vi "GUI_Single Button Pump.vi"() -> ()   [LabVIEW 2011] (continued)
      tunnel: [w32 w122 w128 w148 w153 w159 w162 T20 {"Isolate HPBD"=FALSE, "Core"={"Current VI Reference"=refnum, "Close Panel on Exit?"=FALSE}, "Status Display Array"=[], "Connection URLs"={"Source_URL EC"="", "Target_URL EC"="", "Source_URL LB"="", "Target_URL LB"=""}, "EC Status"={"bits 2"=[], "bits 2"=[], "bits 2"=[], [], "FLOAT NUMBERS 2"=[]}, "EC Status Named"={"EC statusboolarray2"={"Spare 1"=FALSE, "Spare 2"=FALSE, "Spare 3"=FALSE, "Spare 4"=FALSE, "ROUGHING PUMP run opened"=FALSE, "ROUGHING PUMP no fault closed"=FALSE, "BACKING PUMP run opened"=FALSE, "BACKING PUMP no fault closed"=FALSE, "BTL TURBO turbo fault feedback"=FALSE, "BTL TURBO turbo normal feedback"=FALSE, "TARGET 1 TURBO turbo fault feedback"=FALSE, "TARGET 1 TURBO turbo normal feedback"=FALSE, "TARGET 2 TURBO turbo fault feedback"=FALSE, "TARGET 2 TURBO turbo normal feedback"=FALSE, "BTL2 TURBO turbo fault feedback"=FALSE, "BTL2 TURBO turbo normal feedback"=FALSE, "HPD TURBO turbo fault feedback"=FALSE, "HPD TURBO turbo normal feedback"=FALSE, "Spare 5"=FALSE, "Spare 6"=FALSE, "ROUGHING PUMP FLOW SWITCH"=FALSE, "BACKING PUMP FLOW SWITCH"=FALSE, "BTL TURBO FLOW SWITCH"=FALSE, "TARGET 1 TURBO FLOW SWITCH"=FALSE, "TARGET 2 TURBO FLOW SWITCH"=FALSE, "BTL2 TURBO FLOW SWITCH"=FALSE, "HPD TURBO FLOW SWITCH"=FALSE, "Spare 7"=FALSE, "BTL ion gauge on signal"=FALSE, "BTL ion gauge degas signal"=FALSE, "TARGET ion gauge on signal"=FALSE, "TARGET ion gauge degas signal"=FALSE, "BTL2 ion gauge on signal"=FALSE, "BTL2 ion gauge degas signal"=FALSE, "HPD ion gauge on signal"=FALSE, "HPD ion gauge degas signal"=FALSE, "Spare 8"=FALSE, "Spare 9"=FALSE, "Spare 10"=FALSE, "Spare 11"=FALSE, "ROUGHING MANIFOLD VALVE"=FALSE, "BACKING MANIFOLD VALVE"=FALSE, "ROUGHING BACKING CONNECT VALVE"=FALSE, "BTL ROUGHING VALVE"=FALSE, "BTL VENT VALVE"=FALSE, "BTL Turbo Gate Valve"=FALSE, "BTL Turbo Backing Valve"=FALSE, "Roughing Manifold VV"=FALSE, "Backing Manifold VV"=FALSE, "TARGET ROUGHING VALVE"=FALSE, "BTL2 ROUGHING VALVE"=FALSE, "HPD ROUGHING VALVE"=FALSE, "GV BTL-TARGET"=FALSE, "GV TARGET-BTL2"=FALSE, "GV BTL2-HPD"=FALSE, "TARGET VENT VALVE"=FALSE, "BTL2 VENT VALVE"=FALSE, "HPD VENT VALVE"=FALSE, "TARGET  Turbo Gate Valve 1"=FALSE, "TARGET  Turbo Gate Valve 2"=FALSE, "BTL2 Turbo Gate Valve"=FALSE, "HPD  Turbo Gate Valve"=FALSE, "TARGET Turbo Backing Valve 1"=FALSE, "TARGET Turbo Backing Valve 2"=FALSE}, "EC statusboolarray3"={"BTL2 Turbo Backing Valve"=FALSE, "HPD Turbo Backing Valve"=FALSE, "Spare 1"=FALSE, "Spare 2"=FALSE, "Spare 3"=FALSE, "Spare 4"=FALSE, "Spare 5"=FALSE, "Spare 6"=FALSE, "Spare 7"=FALSE, "Spare 8"=FALSE, "Spare 9"=FALSE, "BTL Turbo Vent Valve"=FALSE, "TARGET1 Turbo Vent Valve"=FALSE, "TARGET2 Turbo Vent Valve"=FALSE, "BTL2 Turbo Vent Valve"=FALSE, "HPD Turbo Vent Valve"=FALSE, "Spare 10"=FALSE, "Spare 11"=FALSE, "BTL turbo pump run signal"=FALSE, "TARGET1 turbo pump run signal"=FALSE, "TARGET2 turbo pump run signal"=FALSE, "BTL2 turbo pump run signal"=FALSE, "HPD turbo pump run signal"=FALSE, "Spare 12"=FALSE, "watch dog timer - out"=FALSE, "BTL vented – out"=FALSE, "BTL medvac – out"=FALSE, "BTL hivac – out"=FALSE, "GPM EC - out"=FALSE, "GVM EC - out"=FALSE, "RP EC status - out"=FALSE, "RP LB toggle - out"=FALSE, "GATE ALL - closed out"=FALSE, "Spare 13"=FALSE, "Spare 14"=FALSE, "Spare 15"=FALSE, "Spare 16"=FALSE, "Spare 17"=FALSE, "Spare 18"=FALSE, "Spare 19"=FALSE, "Spare 20"=FALSE, "Spare 21"=FALSE, "Spare 22"=FALSE, "Spare 23"=FALSE, "Spare 24"=FALSE, "Spare 25"=FALSE, "Spare 26"=FALSE, "Spare 27"=FALSE}, "EC statusboolarray1"={"BTL ion gauge on feedback"=FALSE, "BTL ion gauge degas feedback"=FALSE, "TARGET ion gauge on feedback"=FALSE, "TARGET ion gauge degas feedback"=FALSE, "BTL2 ion gauge on feedback"=FALSE, "BTL2 ion gauge degas feedback"=FALSE, "HPD ion gauge on feedback"=FALSE, "HPD ion gauge degas feedback"=FALSE, "Spare 1"=FALSE, "Spare 2"=FALSE, "Spare 3"=FALSE, "Spare 4"=FALSE, "ROUGHING MANIFOLD VALVE opened"=FALSE, "ROUGHING MANIFOLD VALVE closed"=FALSE, "BACKING MANIFOLD VALVE opened"=FALSE, "BACKING MANIFOLD VALVE closed"=FALSE, "ROUGHING BACKING CONNECT VALVE opened"=FALSE, "ROUGHING BACKING CONNECT VALVE closed"=FALSE, "BTL ROUGHING VALVE opened"=FALSE, "BTL ROUGHING VALVE closed"=FALSE, "BTL VENT VALVE opened"=FALSE, "BTL VENT VALVE closed"=FALSE, "BTL Turbo Gate Valve opened"=FALSE, "BTL Turbo Gate Valve closed"=FALSE, "BTL Turbo Backing Valve opened"=FALSE, "BTL Turbo Backing Valve closed"=FALSE, "Roughing Manifold VV opened"=FALSE, "Roughing Manifold VV closed"=FALSE, "Backing Manifold VV opened"=FALSE, "Backing Manifold VV closed"=FALSE, "TARGET ROUGHING VALVE opened"=FALSE, "TARGET ROUGHING VALVE closed"=FALSE, "BTL2 ROUGHING VALVE opened"=FALSE, "BTL2 ROUGHING VALVE closed"=FALSE, "HPD ROUGHING VALVE opened"=FALSE, "HPD ROUGHING VALVE closed"=FALSE, "GV BTL-TARGET opened"=FALSE, "GV BTL-TARGET closed"=FALSE, "GV TARGET-BTL2 opened"=FALSE, "GV TARGET-BTL2 closed"=FALSE, "GV BTL2-HPD opened"=FALSE, "GV BTL2-HPD closed"=FALSE, "TARGET VENT VALVE opened"=FALSE, "TARGET VENT VALVE closed"=FALSE, "BTL2 VENT VALVE opened"=FALSE, "BTL2 VENT VALVE closed"=FALSE, "HPD VENT VALVE opened"=FALSE, "HPD VENT VALVE closed"=FALSE, "TARGET  Turbo Gate Valve 1 opened"=FALSE, "TARGET  Turbo Gate Valve 1 closed"=FALSE, "TARGET  Turbo Gate Valve 2 opened"=FALSE, "TARGET  Turbo Gate Valve 2 closed"=FALSE, "BTL2 Turbo Gate Valve opened"=FALSE, "BTL2 Turbo Gate Valve closed"=FALSE, "HPD  Turbo Gate Valve opened"=FALSE, "HPD  Turbo Gate Valve closed"=FALSE, "TARGET Turbo Backing Valve 1 opened"=FALSE, "TARGET Turbo Backing Valve 1 closed"=FALSE, "TARGET Turbo Backing Valve 2 opened"=FALSE, "TARGET Turbo Backing Valve 2 closed"=FALSE, "BTL2 Turbo Backing Valve opened"=FALSE, "BTL2 Turbo Backing Valve closed"=FALSE, "HPD Turbo Backing Valve opened"=FALSE, "HPD Turbo Backing Valve closed"=FALSE}, "EC statusintegerarray"={"BTL vacuum status word convectron ATM"=0, "TARGET vacuum status word convectron ATM 2"=0, "BTL2 vacuum status word convectron ATM 3"=0, "HPD vacuum status word convectron ATM 4"=0, "Spare 1"=0, "Spare 2"=0, "roughing pump vacuum status word convectron"=0, "backing pump vacuum status word convectron"=0, "roughing manifold vacuum status word convectron"=0, "backing manifold vacuum status word convectron"=0, "BTL Convectron vacuum status word convectron"=0, "TARGET1 Convectron vacuum status word convectron"=0, "TARGET2 Convectron vacuum status word convectron"=0, "BTL2 Convectron vacuum status word convectron"=0, "HPD Convectron vacuum status word convectron"=0, "BTL status word turbo pump"=0, "TARGET1 status word turbo pump"=0, "TARGET2 status word turbo pump"=0, "BTL2 status word turbo pump??"=0, "HPD status word turbo pump"=0, "Spare 3"=0, "Spare 4"=0, "Spare 5"=0, "Spare 6"=0, "BTL CONVECTRON Consolidate"=0, "Spare 7"=0, "Spare 8"=0, "Spare 9"=0, "TARGET Consolidate"=0, "Spare 10"=0, "Spare 11"=0, "Spare 12"=0, "BTL2 Consolidate"=0, "Spare 13"=0, "Spare 14"=0, "Spare 15"=0, "HPD Consolidate"=0, "Spare 16"=0, "Spare 17"=0, "Spare 18"=0, "Spare 19"=0, "Spare 20"=0, "Spare 21"=0, "Spare 22"=0, "Spare 23"=0, "Spare 24"=0, "Spare 25"=0, "Spare 26"=0}, "EC statusfloatarray"={"BTL READING ION GAUGE"=0.0, "TARGET READING ION GAUGE"=0.0, "BTL2 READING ION GAUGE"=0.0, "HPD READING ION GAUGE"=0.0, "Spare 1"=0.0, "Spare 2"=0.0, "Spare 3"=0.0, "Spare 4"=0.0, "roughing pump READING CONVECTRON GAUGE"=0.0, "backing pump READING CONVECTRON GAUGE"=0.0, "roughing manifold READING CONVECTRON GAUGE"=0.0, "backing manifold READING CONVECTRON GAUGE"=0.0, "BTL Convectron READING CONVECTRON GAUGE"=0.0, "TARGET1 READING CONVECTRON GAUGE"=0.0, "TARGET2 READING CONVECTRON GAUGE"=0.0, "BTL2 READING CONVECTRON GAUGE"=0.0, "HPD READING CONVECTRON GAUGE"=0.0, "Spare 5"=0.0, "Spare 6"=0.0, "Spare 7"=0.0, "Spare 8"=0.0, "Spare 9"=0.0, "Spare 10"=0.0, "Spare 11"=0.0}}, "TCPConnection"={"Status TCP Connection EC"=refnum, "Command TCP Connection EC"=refnum, "Status TCP Connection LB"=refnum, "Command TCP Connection LB"=refnum}, "EC Command Cluster"={"boolarray1"={FALSE, FALSE, FALSE, FALSE, FALSE, FALSE, FALSE, FALSE, FALSE, FALSE, FALSE, FALSE, FALSE, FALSE, FALSE, FALSE}, "boolarray2"={FALSE, FALSE, FALSE, FALSE, FALSE, FALSE, FALSE, FALSE, FALSE, FALSE, FALSE, FALSE, FALSE, FALSE, FALSE, FALSE}, "boolarray3"={FALSE, FALSE, FALSE, FALSE, FALSE, FALSE, FALSE, FALSE, FALSE, FALSE, FALSE, FALSE, FALSE, FALSE, FALSE, FALSE}, "boolarray4"={FALSE, FALSE, FALSE, FALSE, FALSE, FALSE, FALSE, FALSE, FALSE, FALSE, FALSE, FALSE, FALSE, FALSE, FALSE, FALSE}}, "EC Command Named"={"EC Command array 1"={"ROUGHING MANIFOLD VALVE"=FALSE, "BACKING MANIFOLD VALVE"=FALSE, "ROUGHING BACKING CONNECT VALVE"=FALSE, "BTL ROUGHING VALVE"=FALSE, "BTL VENT VALVE"=FALSE, "BTL Turbo Gate Valve"=FALSE, "BTL Turbo Backing Valve"=FALSE, "Roughing Manifold VV"=FALSE, "Backing Manifold VV"=FALSE, "TARGET ROUGHING VALVE"=FALSE, "BTL2 ROUGHING VALVE"=FALSE, "HPD ROUGHING VALVE"=FALSE, "GV BTL-TARGET"=FALSE, "GV TARGET-BTL2"=FALSE, "GV BTL2-HPD"=FALSE, "TARGET VENT VALVE"=FALSE}, " EC Command array 2"={"BTL2 VENT VALVE"=FALSE, "HPD VENT VALVE"=FALSE, "TARGET  Turbo Gate Valve 1"=FALSE, "TARGET  Turbo Gate Valve 2"=FALSE, "BTL2 Turbo Gate Valve"=FALSE, "HPD  Turbo Gate Valve"=FALSE, "TARGET Turbo Backing Valve 1"=FALSE, "TARGET Turbo Backing Valve 2"=FALSE, "BTL2 Turbo Backing Valve"=FALSE, "HPD Turbo Backing Valve"=FALSE, "Spare 1"=FALSE, "Spare 2"=FALSE, "ROUGHING PUMP"=FALSE, "BACKING PUMP"=FALSE, "Spare 3"=FALSE, "Spare 4"=FALSE}, "EC Command array 3"={"Spare 1"=FALSE, "Spare 2"=FALSE, "Spare 3"=FALSE, "BTL Turbo Vent Valve"=FALSE, "TARGET1 Turbo Vent Valve"=FALSE, "TARGET2 Turbo Vent Valve"=FALSE, "BTL2 Turbo Vent Valve"=FALSE, "HPD Turbo Vent Valve"=FALSE, "Spare 4"=FALSE, "Spare 5"=FALSE, "GPM"=FALSE, "GVM"=FALSE, "Spare 6"=FALSE, "BTL turbo pump"=FALSE, "TARGET1 turbo pump"=FALSE, "TARGET2 turbo pump"=FALSE}, "EC Command array 4"={"BLT turbo pump"=FALSE, "HPD turbo pump"=FALSE, "Spare 1"=FALSE, "BTL ION GAUGE ion gauge"=FALSE, "BTL ION GAUGE  ion gauge degas"=FALSE, "TARGET ion gauge"=FALSE, "TARGET ion gauge degas"=FALSE, "BTL2 ion gauge"=FALSE, "BTL2 ion gauge degas"=FALSE, "HPD ion gauge"=FALSE, "HPD ion gauge degas"=FALSE, "Spare 2"=FALSE, "Spare 3"=FALSE, "Spare 4"=FALSE, "Spare 5"=FALSE, "Spare 6"=FALSE}}, "LB Status Named"={"LB statusboolarray1"={"COMP ion gauge on feedback"=FALSE, "COMP ion gauge degas feedback"=FALSE, "M123 ion gauge on feedback"=FALSE, "M123 ion gauge degas feedback"=FALSE, "OAP ion gauge on feedback"=FALSE, "OAP ion gauge degas feedback"=FALSE, "Spare 1"=FALSE, "Spare 2"=FALSE, "Spare 3"=FALSE, "Spare 4"=FALSE, "Spare 5"=FALSE, "Spare 6"=FALSE, "ROUGHING MANIFOLD VALVE opened"=FALSE, "ROUGHING MANIFOLD VALVE closed"=FALSE, "BACKING MANIFOLD VALVE opened"=FALSE, "BACKING MANIFOLD VALVE closed"=FALSE, "ROUGHING BACKING CONNECT VALVE opened"=FALSE, "ROUGHING BACKING CONNECT VALVE closed"=FALSE, "COMPRESSOR ROUGHING VALVE opened"=FALSE, "COMPRESSOR ROUGHING VALVE closed"=FALSE, "M123 ROUGHING VALVE opened"=FALSE, "M123 ROUGHING VALVE closed"=FALSE, "BEAMDUMP ROUGHING VALVE opened"=FALSE, "BEAMDUMP ROUGHING VALVE closed"=FALSE, "OAP ROUGHING VALVE opened"=FALSE, "OAP ROUGHING VALVE closed"=FALSE, "GATE VALVE COMP-M123 opened"=FALSE, "GATE VALVE COMP-M123 closed"=FALSE, "GATE VALVE BEAM DUMP opened"=FALSE, "GATE VALVE BEAM DUMP closed"=FALSE, "GATE VALVE M123-OAP opened"=FALSE, "GATE VALVE M123-OAP closed"=FALSE, "GATE VALVE OAP-BTL opened"=FALSE, "GATE VALVE OAP-BTL closed"=FALSE, "COMPRESSOR VENT VALVE opened"=FALSE, "COMPRESSOR VENT VALVE closed"=FALSE, "M123 VENT VALVE opened"=FALSE, "M123 VENT VALVE closed"=FALSE, "BEAMDUMP VENT VALVE opened"=FALSE, "BEAMDUMP VENT VALVE closed"=FALSE, "OAP VENT VALVE opened"=FALSE, "OAP VENT VALVE closed"=FALSE, "COMPRESSOR Turbo Gate Valve opened "=FALSE, "COMPRESSOR Turbo Gate Valve closed"=FALSE, "M123 Turbo Gate Valve opened"=FALSE, "M123 Turbo Gate Valve closed"=FALSE, "OAP Turbo Gate Valve opened"=FALSE, "OAP Turbo Gate Valve closed"=FALSE, "COMPRESSOR Turbo Backing Valve opened"=FALSE, "COMPRESSOR Turbo Backing Valve closed"=FALSE, "M123 Turbo Backing Valve opened"=FALSE, "M123 Turbo Backing Valve closed"=FALSE, "OAP Turbo Backing Valve opened"=FALSE, "OAP Turbo Backing Valve closed"=FALSE, "Roughing Manifold Vent Valve opened"=FALSE, "Roughing Manifold Vent Valve closed"=FALSE, "Spare 7"=FALSE, "Spare 8"=FALSE, "Spare 9"=FALSE, "Spare 10"=FALSE, "RP RUN opened"=FALSE, "RP no FAULT closed"=FALSE, "BP RUN opened"=FALSE, "BP no FAULT closed"=FALSE}, "LB statusboolarray2"={"Spare 1"=FALSE, "Spare 2"=FALSE, "Spare 3"=FALSE, "Spare 4"=FALSE, "ROUGHING PUMP run"=FALSE, "ROUGHING PUMP no fault"=FALSE, "BACKING PUMP run"=FALSE, "BACKING PUMP no fault"=FALSE, "COMP TURBO fault feedback"=FALSE, "COMP TURBO normal feedback"=FALSE, "M123 TURBO fault feedback"=FALSE, "M123 TURBO normal feedback"=FALSE, "OAP TURBO fault feedback"=FALSE, "OAP TURBO normal feedback"=FALSE, "Spare 9"=FALSE, "Spare 10"=FALSE, "Spare 11"=FALSE, "Spare 12"=FALSE, "Spare 13"=FALSE, "Spare 14"=FALSE, "ROUGHING PUMP FLOW SWITCH"=FALSE, "BACKING PUMP FLOW SWITCH"=FALSE, "COMP TURBO FLOW SWITCH"=FALSE, "M123 TURBO FLOW SWITCH"=FALSE, "OAP TURBO FLOW SWITCH"=FALSE, "Spare 15"=FALSE, "Spare 16"=FALSE, "Spare 17"=FALSE, "COMP ion gauge on signal"=FALSE, "COMP ion gauge degas signal"=FALSE, "M123 ion gauge on signal"=FALSE, "M123 ion gauge degas signal"=FALSE, "OAP ion gauge on signal"=FALSE, "OAP ion gauge degas signal"=FALSE, "Spare 18"=FALSE, "Spare 19"=FALSE, "Spare 20"=FALSE, "Spare 21"=FALSE, "Spare 22"=FALSE, "Spare 23"=FALSE, "ROUGHING MANIFOLD VALVE"=FALSE, "BACKING MANIFOLD VALVE"=FALSE, "ROUGHING BACKING CONNECT VALVE"=FALSE, "COMPRESSOR ROUGHING VALVE"=FALSE, "M123 ROUGHING VALVE"=FALSE, "BEAMDUMP ROUGHING VALVE"=FALSE, "OAP ROUGHING VALVE"=FALSE, "GATE VALVE COMP-M123"=FALSE, "GATE VALVE BEAM DUMP"=FALSE, "GATE VALVE M123-OAP"=FALSE, "GATE VALVE OAP-BTL"=FALSE, "COMPRESSOR VENT VALVE"=FALSE, "M123 VENT VALVE"=FALSE, "BEAMDUMP VENT VALVE"=FALSE, "OAP VENT VALVE"=FALSE, "COMPRESSOR Turbo Gate Valve"=FALSE, "M123 Turbo Gate Valve"=FALSE, "OAP Turbo Gate Valve"=FALSE, "COMPRESSOR Turbo Backing Valve"=FALSE, "M123 Turbo Backing Valve"=FALSE, "OAP Turbo Backing Valve"=FALSE, "Spare 24"=FALSE, "Spare 25"=FALSE, "Spare 26"=FALSE}, "LB statusboolarray3"={"Spare 1"=FALSE, "Spare 2"=FALSE, "Spare 3"=FALSE, "Spare 4"=FALSE, "ROUGHING PUMP"=FALSE, "BACKING PUMP"=FALSE, "Spare 5"=FALSE, "Spare 6"=FALSE, "Spare 7"=FALSE, "Spare 8"=FALSE, "Spare 9"=FALSE, "COMP Turbo Vent Valve"=FALSE, "M123 Turbo Vent Valve"=FALSE, "OAP Turbo Vent Valve"=FALSE, "Spare 10"=FALSE, "Spare 11"=FALSE, "Spare 12"=FALSE, "Spare 13"=FALSE, "COMP turbo pump run signal"=FALSE, "M123 turbo pump run signal"=FALSE, "OAP turbo pump run signal"=FALSE, "Spare 14"=FALSE, "Spare 15"=FALSE, "Spare 16"=FALSE, "watch dog timer - out"=FALSE, "GATE OAP-BTL - closed out"=FALSE, "GATE 1 – closed out"=FALSE, "GATE 2 – closed out"=FALSE, "GATE 3,4 – closed out"=FALSE, "GPM LB - out"=FALSE, "GVM LB - out"=FALSE, "RP LB status - out"=FALSE, "RP EC - toggle - out"=FALSE, "Spare 17"=FALSE, "Spare 18"=FALSE, "Spare 19"=FALSE, "Spare 20"=FALSE, "Spare 21"=FALSE, "Spare 22"=FALSE, "Spare 23"=FALSE}, "LB statusintegerarray"={"COMP vacuum status word convectron ATM"=0, "M123 vacuum status word convectron ATM"=0, "OAP vacuum status word convectron ATM"=0, "HPBD vacuum status word convectron ATM"=0, "Spare 1"=0, "Spare 2"=0, "roughing pump vacuum status word convectron"=0, "backing pump vacuum status word convectron"=0, "roughing manifold vacuum status word convectron"=0, "backing manifold vacuum status word convectron"=0, "COMP Convectron vacuum status word convectron"=0, "M123 Convectron vacuum status word convectron"=0, "OAP Convectron vacuum status word convectron"=0, "Spare 3"=0, "Spare 4"=0, "COMP status word turbo pump"=0, "M123 status word turbo pump"=0, "OAP status word turbo pump"=0, "Spare 5"=0, "Spare 6"=0, "Spare 7"=0, "Spare 8"=0, "Spare 9"=0, "Spare 10"=0, "COMP CONVECTRON consloidate"=0, "Spare 11"=0, "Spare 12"=0, "Spare 13"=0, "M123 CONVECTRON consloidate"=0, "Spare 14"=0, "Spare 15"=0, "Spare 16"=0, "OAP CONVECTRON consloidate"=0, "Spare 17"=0, "Spare 18"=0, "Spare 19"=0, "HPBD CONVECTRON consloidate"=0, "Spare 20"=0, "Spare 21"=0, "Spare 22"=0, "Spare 23"=0, "Spare 24"=0, "Spare 25"=0, "Spare 26"=0, "Spare 27"=0, "Spare 28"=0, "Spare 29"=0, "Spare 30"=0}, "LB statusfloatarray"={"COMP READING ION GAUGE"=0.0, "M123 READING ION GAUGE"=0.0, "OAP READING ION GAUGE"=0.0, "Spare 1"=0, "Spare 2"=0, "Spare 3"=0, "Spare 4"=0, "Spare 5"=0, "roughing pump CONVECTRON GAUGE"=0.0, "backing pump CONVECTRON GAUGE"=0.0, "roughing manifold CONVECTRON GAUGE"=0.0, "backing manifold CONVECTRON GAUGE"=0.0, "COMP Convectron CONVECTRON GAUGE"=0.0, "M123 Convectron CONVECTRON GAUGE"=0.0, "OAP Convectron CONVECTRON GAUGE"=0.0, "Spare 6"=0, "Spare 7"=0, "Spare 8"=0, "Spare 9"=0, "Spare 10"=0, "Spare 11"=0, "Spare 12"=0, "Spare 13"=0, "Spare 14"=0}}, "LB Status"={"bits 2"=[], "bits 2"=[], "bits 2"=[], [], "FLOAT NUMBERS 2"=[]}, "LB Command Cluster"={"boolarray1"={FALSE, FALSE, FALSE, FALSE, FALSE, FALSE, FALSE, FALSE, FALSE, FALSE, FALSE, FALSE, FALSE, FALSE, FALSE, FALSE}, "boolarray2"={FALSE, FALSE, FALSE, FALSE, FALSE, FALSE, FALSE, FALSE, FALSE, FALSE, FALSE, FALSE, FALSE, FALSE, FALSE, FALSE}, "boolarray3"={FALSE, FALSE, FALSE, FALSE, FALSE, FALSE, FALSE, FALSE, FALSE, FALSE, FALSE, FALSE, FALSE, FALSE, FALSE, FALSE}, "boolarray4"={FALSE, FALSE, FALSE, FALSE, FALSE, FALSE, FALSE, FALSE, FALSE, FALSE, FALSE, FALSE, FALSE, FALSE, FALSE, FALSE}}, "LB Command Named"={"LB commandarray1"={"ROUGHING MANIFOLD VALVE"=FALSE, "BACKING MANIFOLD VALVE"=FALSE, "ROUGHING BACKING CONNECT VALVE"=FALSE, "COMPRESSOR ROUGHING VALVE"=FALSE, "M123 ROUGHING VALVE"=FALSE, "BEAMDUMP ROUGHING VALVE"=FALSE, "OAP ROUGHING VALVE"=FALSE, "GATE VALVE COMP-M123"=FALSE, "GATE VALVE BEAM DUMP"=FALSE, "GATE VALVE M123-OAP"=FALSE, "GATE VALVE OAP-BTL"=FALSE, "COMPRESSOR VENT VALVE"=FALSE, "M123 VENT VALVE"=FALSE, "BEAMDUMP VENT VALVE"=FALSE, "OAP VENT VALVE"=FALSE, "COMPRESSOR Turbo Gate Valve"=FALSE}, "LB commandarray2"={"M123 Turbo Gate Valve"=FALSE, "OAP Turbo Gate Valve"=FALSE, "COMPRESSOR Turbo Backing Valve"=FALSE, "M123 Turbo Backing Valve"=FALSE, "OAP Turbo Backing Valve"=FALSE, "Roughing Manifold Vent Valve"=FALSE, "Backing Manifold Vent Valve"=FALSE, "Spare 1"=FALSE, "Spare 2"=FALSE, "Spare 3"=FALSE, "Spare 4"=FALSE, "Spare 5"=FALSE, "ROUGHING PUMP"=FALSE, "BACKING PUMP"=FALSE, "Spare 6"=FALSE, "Spare 7"=FALSE}, "LB commandarray3"={"Spare 1"=FALSE, "Spare 2"=FALSE, "Spare 3"=FALSE, "COMP Turbo Vent Valve"=FALSE, "M123 Turbo Vent Valve"=FALSE, "OAP Turbo Vent Valve"=FALSE, "Spare 4"=FALSE, "Spare 5"=FALSE, "Spare 6"=FALSE, "Spare 7"=FALSE, "GPM"=FALSE, "GVM"=FALSE, "Spare 8"=FALSE, "COMP turbo pump"=FALSE, "M123 turbo pump"=FALSE, "OAP turbo pump"=FALSE}, "LB commandarray4"={"Spare 1"=FALSE, "Spare 2"=FALSE, "Spare 3"=FALSE, "COMP ION GAUGE"=FALSE, "COMP ION GAUGE degas"=FALSE, "M123 ION GAUGE"=FALSE, "M123 ION GAUGE degas"=FALSE, "OAP ION GAUGE"=FALSE, "OAP ION GAUGE degas"=FALSE, "Spare 4"=FALSE, "Spare 5"=FALSE, "Spare 6"=FALSE, "Spare 7"=FALSE, "Spare 8"=FALSE, "Spare 9"=FALSE, "Spare 10"=FALSE}}, "VI Refnum"=refnum, "Chamber Selection"={"COMP"=FALSE, "M123"=FALSE, "HPBD"=FALSE, "OAP"=FALSE, "BTL"=FALSE, "TARGET"=FALSE, "BTL2"=FALSE, "HPD"=FALSE}, "GPM Mode"=enum."Complete Global Pump Mode", "Debug Mode?"=FALSE, "State Sanity Check Array"=[], "Critical Failures"={"GPM Exit?"=FALSE}, "Comm Ready?"=FALSE, "Status Reconnect Attempt"=0.0} ("output cluster") w179 w186 w191 w204 w211 w224 w231 w244 w254 w269 w275 w344 w349 w355 w364 w391 w398 w406 w419 w420 w432 w441 w531 w622 w713 w804 w894 w975 w1025 w1087 w1127 w1231 w1284 w1300 w1306 w1310 w1345 w1393 w1398 w1449 w1499 w1522 w1572 w1578 w1600 w1640 w1667 w1706 w1712 w1732 w1751 w1754 w1775 w1797 w1816 w1838 w1843 w1865 w1889 w1914 w1934 w1959 w1983 w2005 w2033 w2053 w2116 w2203 w2222 w2237 w2283] -> w18
      tunnel: w16 -> [w31 _ _ _ _ _ _ _ _ _ _ _ _ _ _ _ _ _ _ _ _ _ _ _ _ _ _ _ _ _ _ _ _ _ _ _ _ _ _ _ _ _ _ _ _ _ _ _ _ _ _ _ _ _ _ _ _ _ _ _ _ _ _ _ _ _ _ _ _ _ _ _ _ _ _ _ _ _ _]
      tunnel: w14 -> [w30 _ _ _ _ _ _ _ _ _ _ _ _ _ _ _ _ _ _ _ _ _ _ _ _ _ _ _ _ _ _ _ _ _ _ _ _ _ _ _ _ _ _ _ _ _ _ _ _ _ _ _ _ _ _ _ _ _ _ _ _ _ _ _ _ _ _ _ _ _ _ _ _ _ _ _ _ _ _]
      tunnel: w13 -> [w29 _ _ _ _ _ _ _ _ _ _ _ _ _ _ _ _ _ _ _ _ _ _ _ _ _ _ _ _ w445 w535 w626 w717 w808 w898 w984 w1032 w1090 w1138 w1242 _ _ _ _ w1360 _ w1410 w1461 _ w1535 _ _ w1612 _ w1677 _ _ w1743 _ w1767 w1788 _ w1829 _ _ w1881 _ w1918 w1951 _ w1998 w2022 _ _ w2126 _ _ w2246 _]
      tunnel: w12 -> [_ _ _ _ _ _ _ _ _ _ _ _ _ _ _ _ _ _ _ _ _ _ _ _ _ _ _ _ _ w443 w533 w624 w715 w806 w896 w982 w1020 w1078 w1129 w1235 _ _ _ _ w1349 _ w1400 w1451 _ w1525 _ _ w1601 _ w1669 _ _ w1737 _ w1756 w1778 _ w1819 _ _ w1871 _ w1917 w1942 _ w1981 w2012 _ _ w2120 _ _ w2240 _]
      tunnel: [_ _ _ _ _ _ _ _ _ _ _ _ _ _ _ _ _ _ FALSE _ _ _ _ _ FALSE FALSE FALSE _ TRUE TRUE TRUE TRUE TRUE TRUE TRUE TRUE TRUE TRUE TRUE TRUE TRUE TRUE _ _ _ _ _ _ _ _ _ _ _ _ _ _ _ _ _ _ _ _ _ _ _ _ _ _ _ _ _ _ _ _ _ _ _ _ _] -> w9
      frame "", "Idle" {
        n8 = event shown="[0] Timeout" {
          selector: w30 -> [_ _ _ _ _ _]
          dyn-events: _ -> [_ _ _ _ _ _]
          timeout: w31 -> [_ _ _ _ _ _]
          tunnel: w37 -> [w38 w46 w52 w68 w93 w121]
          tunnel: [w38 w47 w51 w69 w93 w120] -> w36
          tunnel: w35 -> [w39 w45 w49 w60 w89 w118]
          tunnel: [w40 w44 w50 w57 w94 w119] -> w34
          tunnel: w33 -> [w40 w44 w50 w58 w95 w119]
          tunnel: [w39 w45 w49 w59 w92 w118] -> w32
          tunnel: w29 -> [_ _ _ _ _ _]
          event Timeout {
            n9 = event-data() -> ()  [unwired: 1 in, 1 out]
          }
          event "Pump": Value Change {
            n10 = event-data() -> ("CtlRef"=w43:refnum<vi>)  [unwired: 1 in, 5 out]
            n11 = property class="Bool"(reference=w43, "DisabledEnum"=T18."Disabled and Grayed Out" ("Disabled")) -> ()  [unwired: 1 in, 2 out]
            n12 = call <vilib>:"Add State(s) to Queue__jki_lib_state_machine.vi"("State(s) in Front (\"\")"="Main: Check GPM GVM Mode Status>>PreCheck", "State(s) in (\"\")"=w46) -> ("States Out"=w47:string)  [unwired: 13 in]
          }
          event "OK": Value Change {
            # "Exit Button Value Change (pressed) Event\n(this executes Macro: Exit to terminate the VI)"
            n13 = event-data() -> ()  [unwired: 1 in, 1 out]
            n14 = call <vilib>:"Add State(s) to Queue__jki_lib_state_machine.vi"("State(s) in Front (\"\")"="Macro: Exit", "State(s) in (\"\")"=w52) -> ("States Out"=w51:string)  [unwired: 13 in]
          }
          event User Event {
            n15 = event-data() -> ("Error Action"=w53:T16, "Error Codes"=w56:T17, "Status Array"=w62:string[])  [unwired: 1 in, 4 out]
            n16 = Unbundle By Name(w60) -> ("Status Display Array"=w64:string[])
            n17 = call <userlib>:"Get Strings from Enum__ogtk.vi"("Enum"=w56) -> ("String Value"=w67:string)  [unwired: 7 in, 3 out]
            n18 = Scan From String(format string="%d", input string=w67, error in=w58, default 1=0) -> (error out=w57:errorcluster, output 1=w63:i32)  [unwired: 1 in, 2 out]
            n19 = call "RemoveStatus Display Messages.vi"("Numeric"=w63, "Status Display Array"=w64) -> ("array w/ subset deleted"=w61:string[])  [unwired: 9 in]
            n20 = case shown="\"004-Check Chamber Pressures\"" w56 {
              tunnel: [w71 "Some of the Turbo Gate Valves are Open" ("Display Message") w77 w81] -> w54
              tunnel: w53 -> [w70 _ w76 w82]
              frame "001-GPM and GVM conditions", Default {
                # "Add Display states here"
                n21 = case shown="\"Add\", Default" w70 {
                  tunnel: ["GPM Mode is currently unavailable " ("Display Message") ""] -> w71
                  frame "Add", Default {
                    n22 = property on="Pump" class="Bool"("DisabledEnum"=T18."Disabled and Grayed Out" ("Disabled")) -> ()  [unwired: 2 in, 2 out]
                  }
                  frame "Remove" {
                  }
                }
              }
              frame "002-Turbo gate valve status" {
              }
              frame "003-Chamber Gate Valve Status" {
                n23 = case shown="\"Add\", Default" w76 {
                  tunnel: ["Gate Valve between Compressor Chamber and \nM123 is Open. Please close this gate valve to continue" ("Display Message") ""] -> w77
                  frame "Add", Default {
                    n24 = property on="Pump" class="Bool"("DisabledEnum"=T18."Disabled and Grayed Out" ("Disabled")) -> ()  [unwired: 2 in, 2 out]
                  }
                  frame "Remove" {
                  }
                }
              }
              frame "004-Check Chamber Pressures" {
                n25 = case shown="\"Remove\"" w82 {
                  tunnel: ["GPM Mode is NOT Available.\nSome of the chambers are under vacuum.\nPlease Vent to have GPM mode available" ("Display Message") "" ("Display Message")] -> w81
                  frame "Add", Default {
                  }
                  frame "Remove" {
                  }
                }
              }
            }
            n26 = case shown="\"Add\", Default" w53 {
              tunnel: w62 -> [w87 _]
              tunnel: w61 -> [w86 w88]
              tunnel: [w85 w88] -> w55
              frame "Add", Default {
                n27 = Build Array (concatenate)(w86, w87) -> (w85:string[])
              }
              frame "Remove" {
              }
            }
            n28 = property on="Errors/Warnings" class="LstBox (strict)"("Item Names"=w55) -> ()  [unwired: 2 in, 2 out]
            n29 = Bundle By Name(cluster=w60, "Status Display Array"=w55) -> (w59:T20)
            n30 = call <vilib>:"Add State(s) to Queue__jki_lib_state_machine.vi"("State(s) in (\"\")"=w68) -> ("States Out"=w69:string)  [unwired: 14 in]
            n31 = property on="Display Message" class="Str"("Value"=w54) -> ()  [unwired: 2 in, 2 out]
          }
          event User Event {
            n32 = event-data() -> ("vi path"=w96:path, "Message"=w90:string)  [unwired: 1 in, 4 out]
            n33 = stacked-sequence {
              tunnel: w96 -> [_ w115]
              tunnel: w95 -> [_ w113]
              tunnel: [_ w110] -> w94
              tunnel: [_ w107] -> w91
              tunnel: w90 -> [_ w106]
              tunnel: w89 -> [w99 _]
              frame #0 {
                n34 = Unbundle By Name(w99) -> ("VI Refnum"=w97:refnum<vi>)
                n35 = Not A Number/Path/Refnum?(number/path/refnum=w97) -> (NaN/Path/Refnum?=w98:bool)
                n36 = case shown="False" w98 {
                  tunnel: w97 -> [w100 _]
                  frame False {
                    n37 = invoke class="VI" method="Abort VI"(reference=w100) -> (reference out=w101:refnum<vi>, error out=w102:errorcluster)  [unwired: 2 in, 1 out]
                    n38 = case shown="No Error" w102 {
                      selector: w102 -> [w104 _]
                      tunnel: w101 -> [w105 _]
                      frame No Error {
                        n39 = Close Reference(reference=w105, error in (no error)=w104) -> (error out=w103:errorcluster)
                        n40 = invoke on="User Input Panel" class="SubPnl" method="Remove VI"(error in=w103) -> ()  [unwired: 2 in, 3 out]
                      }
                      frame Error {
                      }
                    }
                  }
                  frame True {
                  }
                }
              }
              frame #1 {
                n41 = Open VI Reference(vi path=w115, error in (no error)=w113) -> (vi reference=w108:refnum<vi>, error out=w112:errorcluster)  [unwired: 4 in]
                n42 = invoke on="User Input Panel" class="SubPanel" method="Insert VI"(error in=w112, "VI Ref"=w108) -> (error out=w111:errorcluster)  [unwired: 2 in, 3 out]
                n43 = invoke class="VI" method="Ctrl Val.Set"(reference=w108, "Control Name"="Message", "Value"=w106) -> (reference out=w107:refnum<vi>)  [unwired: 2 in, 4 out]
                n44 = invoke class="VI" method="Run VI"(reference=w107, error in=w111, "Wait until done"=FALSE ("Wait Until Done")) -> (error out=w110:errorcluster)  [unwired: 2 in, 4 out]
              }
            }
            n45 = Bundle By Name(cluster=w89, "VI Refnum"=w91) -> (w92:T20)
          }
          event Panel Close? {
            # "Discard the event because we'll close the front panel ourselves in Macro: Exit"
            # "Close Panel button (pressed) Event\n(this executes Macro: Exit to terminate the VI)"
            n46 = event-data() -> ()  [unwired: 1 in, 1 out]
            n47 = call <vilib>:"Add State(s) to Queue__jki_lib_state_machine.vi"("State(s) in Front (\"\")"="Macro: Exit", "State(s) in (\"\")"=w121) -> ("States Out"=w120:string)  [unwired: 13 in]
            n48 = event-data("Discard?"=TRUE) -> ()  [unwired: 1 in, 1 out]
          }
        }
      }
      frame "---------- Core ----------" {
        # "Do not put any code in this frame.\n(it is a separator no-op)"
        n49 = call <vilib>:"Add State(s) to Queue__jki_lib_state_machine.vi"("State(s) in (\"\")"=w125) -> ("States Out"=w124:string)  [unwired: 14 in]
      }
      frame Default {
        w135 = 42 items=["No error", "Argument error", "Memory is full", "Out of zone", "End of file", "File already open", "Generic file I/O error", "File not found", "File permission error", "Disk is full", "Duplicate path", "Too many files open", "System feature not enabled", "Resource file not found", "Cannot add resource", "Resource not found", "Image not found", "Image memory error", "Pen does not exist", "Config type invalid", "Config token not found", "Config parse error", "Config memory error", "Bad external code format", "Bad external code offset", "External code not present", "Null window", "Destroy window error", "Null menu", "Print aborted", "Bad print record", "Print driver error", "Windows error during printing", "Memory error during printing", "Print dialog error", "Generic print error", "Invalid device refnum", "Device not found", "Device parameter error", "Device unit error", "Cannot open device", "Device call aborted", "Generic error", "Cancelled by user", "Object ID too low", "Object ID too high", "Object not in heap", "Unknown heap", "Unknown object (invalid DefProc)", "Unknown object (DefProc not in table)", "Message out of range", "Invalid (null) method", "Unknown message", "Manager call not supported", "Bad address", "Network operation in progress", "Network operation timed out", "Connection is busy", "Network attribute not supported", "Network error", "Address in use", "System out of memory", "Connection aborted", "Connection refused", "Not connected", "Already connected", "Connection closed", "Initialization error (interapplication manager)", "Bad occurrence", "Wait on unbound occurrence handler", "Occurrence queue overflow", "Datalog type conflict", "Unused", "Unrecognized type (interapplication manager)", "Memory corrupt", "Failed to make temporary DLL", "Old CIN version", "Drag socket not found", "Failed to load drop-object", "Failed to register OLE object", "Failed to release OLE object", "Format specifier type mismatch", "Unknown format specifier", "Too few format specifiers", "Too many format specifiers", "Scan failed", "Newer CIN version", "Error converting to variant", "Runtime menu error", "Password tampered", "Variant attribute not found", "Incompatible variant data type", "Event data is not available", "Event Store is not present", "Occurrence is not found", "Event Queue is not created", "Event info is not available", "Refnum passed is NULL", "Error retrieving Class GUID", "Error retrieving CoClass GUID", "Error retrieving TypeLib GUID.", "Bad built application magic bytes.", "Specific driver is different from the specific driver associated with the Logical Name.", "There is no session opened to the class driver.", "Max Error", "MAX - Error with config objects", "MAX - Error loading configuration", "MAX - Group not supported"]
        # "Current State"
        # "Do not delete, rename, or modify this frame.\n(this is used to capture unhandled states and typos)"
        # "Handle mistyped state name (developer tool)"
        n50 = Format Into String(format string="Software Exception: Unhandled State \"%s\"." ("message"), error in=w131, w126) -> (resulting string=w134:string, error out=w133:errorcluster)  [unwired: 1 in]
        n51 = call <vilib>:"Error Cluster From Error Code.vi"("show call chain? (False)"=TRUE, "error in (no error)"=w133, "error message (\"\")"=w134, "error code (0)"=w135) -> ("error out"=w132:errorcluster)  [unwired: 5 in]
        n52 = call <vilib>:"Add State(s) to Queue__jki_lib_state_machine.vi"("State(s) in (\"\")"=w130) -> ("States Out"=w129:string)  [unwired: 14 in]
      }
      frame "Initialize Core Data" {
        # "Do not delete, rename, or modify this frame.\n(this is used to determine panel behavior on exit)"
        # "originally closed?"
        # "exe?"
        # "If panel starts closed or is an EXE, then close it when we exit"
        n53 = property class="VI"() -> ("Front Panel.Open"=w146:bool)  [unwired: 2 in, 2 out]
        n54 = property class="App"() -> ("App.Kind"=w145:T19)  [unwired: 2 in, 2 out]
        n55 = control-ref of="Current VI Reference"() -> (w139:refnum<vi>)
        n56 = Not(x=w146) -> (.not. x?=w143:bool)
        n57 = Equal?(x=w145, y=T19."Run Time System" ("Application:Kind")) -> (x = y?=w142:bool)
        n58 = Or(x=w143, y=w142) -> (x .or. y?=w140:bool)
        n59 = Bundle By Name(cluster=w141, "Core.Current VI Reference"=w139, "Core.Close Panel on Exit?"=w140, "Debug Mode?"="Debug Mode?", "Status Reconnect Attempt"=0.0) -> (w148:T20)
        n60 = call <vilib>:"Add State(s) to Queue__jki_lib_state_machine.vi"("State(s) in (\"\")"=w150) -> ("States Out"=w149:string)  [unwired: 14 in]
      }
      frame "Error Handler" {
        # "Unhandled Error -- Display it"
        # "Handle any errors here.\nYou can also output any states to clean-up after errors occur"
        # "Clear error"
        n61 = call <vilib>:"General Error Handler.vi"("error in (no error)"=w152) -> ()  [unwired: 10 in, 5 out]
        n62 = call <vilib>:"Add State(s) to Queue__jki_lib_state_machine.vi"("State(s) in Front (\"\")"="/* Post Error States", "State(s) in (\"\")"=w156) -> ("States Out"=w155:string)  [unwired: 13 in]
      }
      frame "Exit" {
        # "Do not put any code in this frame.\n(No errors that occur here will be handled.)"
        n63 = call <vilib>:"Add State(s) to Queue__jki_lib_state_machine.vi"("State(s) in (\"\")"=w161) -> ("States Out"=w160:string)  [unwired: 14 in]
      }
      frame "---------- Data ----------" {
        # "Do not put any code in this frame.\n(It is a separator no-op. You can make a copy of this frame to create a new Data frame)"
        n64 = call <vilib>:"Add State(s) to Queue__jki_lib_state_machine.vi"("State(s) in (\"\")"=w165) -> ("States Out"=w164:string)  [unwired: 14 in]
      }
      frame "Data: Initialize" {
        # "Initialize the shift-register data, here.\n(data names are defined by what you wire into the bundle function)"
        n65 = call "DataInit.vi"() -> ()  [unwired: 11 in, 1 out]
        n66 = call <vilib>:"Add State(s) to Queue__jki_lib_state_machine.vi"("State(s) in (\"\")"=w169) -> ("States Out"=w168:string)  [unwired: 14 in]
      }
      frame "Data: Cleanup" {
        # "Cleanup any data and references, here.\n(this is called automatically, by the Macro: Exit)"
        n67 = Unbundle By Name(w179) -> ("Core.Current VI Reference"=w181:refnum<vi>, "TCPConnection.Status TCP Connection EC"=w173:refnum<k5>, "TCPConnection.Command TCP Connection EC"=w172:refnum<k5>, "TCPConnection.Status TCP Connection LB"=w171:refnum<k5>, "TCPConnection.Command TCP Connection LB"=w170:refnum<k5>)
        n68 = TCP Close Connection(connection ID=w173, error in (no error)=w175) -> (error out=w177:errorcluster)  [unwired: 1 in, 1 out]
        n69 = TCP Close Connection(connection ID=w172, error in (no error)=w177) -> (error out=w176:errorcluster)  [unwired: 1 in, 1 out]
        n70 = TCP Close Connection(connection ID=w171, error in (no error)=w176) -> (error out=w178:errorcluster)  [unwired: 1 in, 1 out]
        n71 = TCP Close Connection(connection ID=w170, error in (no error)=w178) -> (error out=w174:errorcluster)  [unwired: 1 in, 1 out]
        n72 = Close Reference(reference=w181, error in (no error)=w174) -> (error out=w180:errorcluster)
        n73 = call <vilib>:"Add State(s) to Queue__jki_lib_state_machine.vi"("State(s) in (\"\")"=w183) -> ("States Out"=w182:string)  [unwired: 14 in]
      }
      frame "---------Connection------------" {
      }
      frame "Connection: Init Status Connection EC" {
        # "Initialize the shift-register data, here.\n(data names are defined by what you wire into the bundle function)"
        n74 = Unbundle By Name(w192) -> ("Connection URLs.Source_URL EC"=w193:string)
        n75 = TCP Open Connection(address=w193, remote port or service name=u16 2447, timeout ms (60000)=14000 ("ms timeout (10000)"), error in (no error)=w189) -> (connection ID=w190:refnum<k5>, error out=w188:errorcluster)  [unwired: 1 in]
        n76 = case shown="Error" w188 {
          tunnel: ["" "Connection: Close Status Connection EC" ("State(s) in Front (\"\")")] -> w187
          frame No Error {
          }
          frame Error {
          }
        }
        n77 = Bundle By Name(cluster=w192, "TCPConnection.Status TCP Connection EC"=w190) -> (w191:T20)
        n78 = call <vilib>:"Add State(s) to Queue__jki_lib_state_machine.vi"("State(s) in Front (\"\")"=w187, "State(s) in (\"\")"=w197) -> ("States Out"=w196:string)  [unwired: 13 in]
      }
      frame "Connection: Close Status Connection EC" {
        # "Initialize the shift-register data, here.\n(data names are defined by what you wire into the bundle function)"
        n79 = Unbundle By Name(w204) -> ("TCPConnection.Status TCP Connection EC"=w203:refnum<k5>)
        n80 = TCP Close Connection(connection ID=w203, error in (no error)=w202) -> (error out=w201:errorcluster)  [unwired: 1 in, 1 out]
        n81 = call <vilib>:"Add State(s) to Queue__jki_lib_state_machine.vi"("State(s) in Front (\"\")"="Connection: Init Status Connection EC" ("State(s) in Front (\"\")"), "State(s) in (\"\")"=w206) -> ("States Out"=w205:string)  [unwired: 13 in]
      }
      frame "Connection: Init Command Connection EC" {
        # "Initialize the shift-register data, here.\n(data names are defined by what you wire into the bundle function)"
        n82 = Unbundle By Name(w212) -> ("Connection URLs.Target_URL EC"=w213:string)
        n83 = TCP Open Connection(address=w213, remote port or service name=u16 2448, timeout ms (60000)=6000 ("ms timeout (10000)"), error in (no error)=w209) -> (connection ID=w210:refnum<k5>, error out=w208:errorcluster)  [unwired: 1 in]
        n84 = case shown="No Error" w208 {
          tunnel: ["" "Connection: Close Command Connection EC" ("State(s) in Front (\"\")")] -> w207
          frame No Error {
          }
          frame Error {
          }
        }
        n85 = Bundle By Name(cluster=w212, "TCPConnection.Command TCP Connection EC"=w210) -> (w211:T20)
        n86 = call <vilib>:"Add State(s) to Queue__jki_lib_state_machine.vi"("State(s) in Front (\"\")"=w207, "State(s) in (\"\")"=w217) -> ("States Out"=w216:string)  [unwired: 13 in]
      }
      frame "Connection: Close Command Connection EC" {
        # "Initialize the shift-register data, here.\n(data names are defined by what you wire into the bundle function)"
        n87 = Unbundle By Name(w224) -> ("TCPConnection.Command TCP Connection EC"=w223:refnum<k5>)
        n88 = TCP Close Connection(connection ID=w223, error in (no error)=w222) -> (error out=w221:errorcluster)  [unwired: 1 in, 1 out]
        n89 = call <vilib>:"Add State(s) to Queue__jki_lib_state_machine.vi"("State(s) in Front (\"\")"="Connection: Init Command Connection EC" ("State(s) in Front (\"\")"), "State(s) in (\"\")"=w226) -> ("States Out"=w225:string)  [unwired: 13 in]
      }
      frame "Connection: Init Status Connection LB" {
        # "Initialize the shift-register data, here.\n(data names are defined by what you wire into the bundle function)"
        n90 = Unbundle By Name(w232) -> ("Connection URLs.Source_URL LB"=w233:string)
        n91 = TCP Open Connection(address=w233, remote port or service name=u16 2447, timeout ms (60000)=14000 ("ms timeout (10000)"), error in (no error)=w229) -> (connection ID=w230:refnum<k5>, error out=w228:errorcluster)  [unwired: 1 in]
        n92 = Bundle By Name(cluster=w232, "TCPConnection.Status TCP Connection LB"=w230) -> (w231:T20)
        n93 = case shown="No Error" w228 {
          tunnel: ["" "Connection: Close Status Connection LB" ("State(s) in Front (\"\")")] -> w227
          frame No Error {
          }
          frame Error {
          }
        }
        n94 = call <vilib>:"Add State(s) to Queue__jki_lib_state_machine.vi"("State(s) in Front (\"\")"=w227, "State(s) in (\"\")"=w237) -> ("States Out"=w236:string)  [unwired: 13 in]
      }
      frame "Connection: Close Status Connection LB" {
        # "Initialize the shift-register data, here.\n(data names are defined by what you wire into the bundle function)"
        n95 = Unbundle By Name(w244) -> ("TCPConnection.Status TCP Connection LB"=w243:refnum<k5>)
        n96 = TCP Close Connection(connection ID=w243, error in (no error)=w242) -> (error out=w241:errorcluster)  [unwired: 1 in, 1 out]
        n97 = call <vilib>:"Add State(s) to Queue__jki_lib_state_machine.vi"("State(s) in Front (\"\")"="Connection: Init Status Connection LB" ("State(s) in Front (\"\")"), "State(s) in (\"\")"=w246) -> ("States Out"=w245:string)  [unwired: 13 in]
      }
      frame "Connection: Init Command Connection LB" {
        # "Initialize the shift-register data, here.\n(data names are defined by what you wire into the bundle function)"
        n98 = Unbundle By Name(w255) -> ("Connection URLs.Target_URL LB"=w256:string)
        n99 = TCP Open Connection(address=w256, remote port or service name=u16 2448, timeout ms (60000)=6000 ("ms timeout (10000)"), error in (no error)=w252) -> (connection ID=w253:refnum<k5>, error out=w251:errorcluster)  [unwired: 1 in]
        n100 = case shown="No Error" w251 {
          tunnel: ["" "Connection: Close Command Connection LB" ("State(s) in Front (\"\")")] -> w250
          tunnel: [TRUE FALSE] -> w247
          frame No Error {
          }
          frame Error {
          }
        }
        n101 = Bundle By Name(cluster=w255, "TCPConnection.Command TCP Connection LB"=w253, "Comm Ready?"=w247) -> (w254:T20)
        n102 = call <vilib>:"Add State(s) to Queue__jki_lib_state_machine.vi"("State(s) in Front (\"\")"=w250, "State(s) in (\"\")"=w260) -> ("States Out"=w259:string)  [unwired: 13 in]
        n103 = call "MID-VAC Timer.vi"("TO sec (Start timer)"=1.0, "Action"=timerAction_typdef."Start Timer") -> ()  [unwired: 9 in, 1 out]
      }
      frame "Connection: Close Command Connection LB" {
        # "Initialize the shift-register data, here.\n(data names are defined by what you wire into the bundle function)"
        n104 = Unbundle By Name(w269) -> ("TCPConnection.Command TCP Connection LB"=w268:refnum<k5>)
        n105 = TCP Close Connection(connection ID=w268, error in (no error)=w267) -> (error out=w266:errorcluster)  [unwired: 1 in, 1 out]
        n106 = call <vilib>:"Add State(s) to Queue__jki_lib_state_machine.vi"("State(s) in Front (\"\")"="Connection: Init Command Connection LB" ("State(s) in Front (\"\")"), "State(s) in (\"\")"=w271) -> ("States Out"=w270:string)  [unwired: 13 in]
      }
      frame "Command: Get Status" {
        n107 = Unbundle By Name(w276) -> ("TCPConnection.Status TCP Connection EC"=w285:refnum<k5>, "TCPConnection.Status TCP Connection LB"=w284:refnum<k5>, "Debug Mode?"=w279:bool)
        n108 = case shown="False" w279 {
          tunnel: w285 -> [w298 _]
          tunnel: w284 -> [w296 _]
          tunnel: w276 -> [w293 w343]
          tunnel: w274 -> [w292 _]
          tunnel: [w286 w340] -> w281
          tunnel: [w288 ""] -> w272
          frame False {
            n109 = call "GetStatus LB.vi"("error in (no error)"=w292, "TCP Network Connection in"=w296) -> ("error out"=w290:errorcluster, "Status"=w294:T26)  [unwired: 8 in]
            n110 = call "GetStatus EC.vi"("error in (no error)"=w292, "TCP Network Connection in"=w298) -> ("error out"=w291:errorcluster, "Status"=w297:T26)  [unwired: 8 in]
            n111 = case shown="No Error" w291 {
              tunnel: w293 -> [w337 w338]
              tunnel: w297 -> [w336 _]
              tunnel: [w325 w338] -> w295
              frame No Error {
                n112 = Unbundle(w336) -> ("bits 2"=w331:bool[], "bits 2"=w333:bool[], "bits 2"=w335:bool[], w329:i32[], "FLOAT NUMBERS 2"=w327:sgl[])
                n113 = Array To Cluster(array=w333) -> (cluster=w332:T27)
                n114 = Array To Cluster(array=w327) -> (cluster=w326:T28)
                n115 = Array To Cluster(array=w331) -> (cluster=w330:T27)
                n116 = Array To Cluster(array=w335) -> (cluster=w334:T29)
                n117 = Array To Cluster(array=w329) -> (cluster=w328:T30)
                n118 = Bundle By Name(cluster=w337, "EC Status"=w336, "EC Status Named.EC statusboolarray1"=w330, "EC Status Named.EC statusboolarray2"=w332, "EC Status Named.EC statusboolarray3"=w334, "EC Status Named.EC statusintegerarray"=w328, "EC Status Named.EC statusfloatarray"=w326) -> (w325:T20)
              }
              frame Error {
              }
            }
            n119 = case shown="No Error" w290 {
              tunnel: w295 -> [w323 w324]
              tunnel: [w322 w324] -> w287
              tunnel: w294 -> [w311 _]
              frame No Error {
                n120 = Unbundle(w311) -> ("bits 2"=w317:bool[], "bits 2"=w319:bool[], "bits 2"=w321:bool[], w315:i32[], "FLOAT NUMBERS 2"=w313:sgl[])
                n121 = Array To Cluster(array=w319) -> (cluster=w318:T27)
                n122 = Array To Cluster(array=w313) -> (cluster=w312:T28)
                n123 = Array To Cluster(array=w317) -> (cluster=w316:T27)
                n124 = Array To Cluster(array=w321) -> (cluster=w320:T31)
                n125 = Array To Cluster(array=w315) -> (cluster=w314:T30)
                n126 = Bundle By Name(cluster=w323, "LB Status"=w311, "LB Status Named.LB statusboolarray1"=w316, "LB Status Named.LB statusboolarray2"=w318, "LB Status Named.LB statusboolarray3"=w320, "LB Status Named.LB statusintegerarray"=w314, "LB Status Named.LB statusfloatarray"=w312) -> (w322:T20)
              }
              frame Error {
              }
            }
            n127 = Merge Errors(w291, w290) -> (w289:errorcluster)
            n128 = case shown="Error" w289 {
              tunnel: w287 -> [w299 w307]
              tunnel: ["" w308] -> w288
              tunnel: w287 -> [_ w306]
              tunnel: [w299 w304] -> w286
              frame No Error {
              }
              frame Error {
                # "Reinit connections on error\nreturn to get Status"
                n129 = Unbundle By Name(w307) -> ("Status Reconnect Attempt"=w303:dbl)
                n130 = Greater?(x=w303, y=5.0) -> (0:w301:bool)
                n131 = case shown="False" w301 {
                  tunnel: ["Connection: Close Status Connection LB\nConnection: Close Status Connection EC\nCommand: Get Status" "Macro: Exit"] -> w308
                  frame False {
                  }
                  frame True {
                    # "TODO: Add exit msg"
                    # "5 attempts, exit"
                  }
                }
                n132 = Increment(x=w303) -> (x+1=w305:dbl)
                n133 = Bundle By Name(cluster=w306, "Status Reconnect Attempt"=w305) -> (w304:T20)
              }
            }
          }
          frame True {
            n134 = Bundle By Name(cluster=w343, "LB Status Named"="LB Status Named", "EC Status Named"="EC Status Named") -> (w340:T20)
          }
        }
        n135 = Unbundle By Name(w281) -> ("LB Status Named.LB statusboolarray3.GPM LB - out"=w282:bool, "EC Status Named.EC statusboolarray3.GPM EC - out"=w283:bool)
        n136 = Or(x=w282, y=w283) -> (x .or. y?=w280:bool)
        n137 = Bundle By Name(cluster=w281, "Critical Failures.GPM Exit?"=w280) -> (w275:T20)
        n138 = call <vilib>:"Add State(s) to Queue__jki_lib_state_machine.vi"("State(s) in Front (\"\")"=w272, "State(s) in (\"\")"=w277) -> ("States Out"=w278:string)  [unwired: 13 in]
      }
      frame "---------- UI ----------" {
        # "Do not put any code in this frame.\n(It is a separator no-op. You can make a copy of this frame to create a new UI frame)"
        n139 = call <vilib>:"Add State(s) to Queue__jki_lib_state_machine.vi"("State(s) in (\"\")"=w347) -> ("States Out"=w346:string)  [unwired: 14 in]
      }
      frame "UI: Initialize" {
        # "Initialize the User Interface, here.\n(this is called automatically, by the Macro: Init)"
        n140 = call <vilib>:"Add State(s) to Queue__jki_lib_state_machine.vi"("State(s) in (\"\")"=w351) -> ("States Out"=w350:string)  [unwired: 14 in]
      }
      frame "UI: Cursor Set" {
        # "Argument"
        # "Set and Unset Cursor Busy.\n(Usage: \"UI: Cursor Set >> Busy|Idle\")"
        n141 = case shown="\"Idle\", Default" w352 {
          tunnel: w354 -> [w359 w361]
          tunnel: [w358 w360] -> w353
          frame "Idle", Default {
            n142 = call <vilib>:"Unset Busy.vi"("error in (no error)"=w359) -> ("error out"=w358:errorcluster)  [unwired: 10 in]
          }
          frame "Busy" {
            n143 = call <vilib>:"Set Busy.vi"("error in (no error)"=w361) -> ("error out"=w360:errorcluster)  [unwired: 9 in, 1 out]
          }
        }
        n144 = call <vilib>:"Add State(s) to Queue__jki_lib_state_machine.vi"("State(s) in (\"\")"=w357) -> ("States Out"=w356:string)  [unwired: 14 in]
      }
      frame "UI: Front Panel State" {
        # "Argument"
        # "Set Front Panel Open or Closed\n(Usage: \"UI: Front Panel State >> Open|Close\")"
        n145 = Unbundle By Name(w364) -> ("Core.Current VI Reference"=w363:refnum<vi>)
        n146 = case shown="\"Open\", Default" w362 {
          tunnel: w366 -> [w372 w385]
          tunnel: [w374 w386] -> w365
          tunnel: w363 -> [w373 w383]
          frame "Open", Default {
            n147 = property class="VI"(reference=w373, error in=w372) -> (reference out=w370:refnum<vi>, error out=w371:errorcluster, "Front Panel.Open"=w369:bool)
            n148 = case shown="False" w369 {
              tunnel: [w377 w380] -> w374
              tunnel: w371 -> [w376 w380]
              tunnel: w370 -> [w375 _]
              frame False {
                n149 = invoke class="VI" method="FP.Open"(reference=w375, error in=w376, "Activate"=TRUE, "State"=T23."Standard") -> (error out=w377:errorcluster)  [unwired: 1 in, 4 out]
              }
              frame True {
              }
            }
          }
          frame "Close" {
            n150 = property class="VI"(reference=w383, error in=w385) -> (reference out=w382:refnum<vi>, error out=w384:errorcluster, "Front Panel.Open"=w381:bool)
            n151 = case shown="True" w381 {
              tunnel: [w387 w390] -> w386
              tunnel: w384 -> [w387 w389]
              tunnel: w382 -> [_ w388]
              frame False {
              }
              frame True {
                n152 = invoke class="VI" method="FP.Close"(reference=w388, error in=w389) -> (error out=w390:errorcluster)  [unwired: 1 in, 2 out]
              }
            }
          }
        }
        n153 = call <vilib>:"Add State(s) to Queue__jki_lib_state_machine.vi"("State(s) in (\"\")"=w368) -> ("States Out"=w367:string)  [unwired: 14 in]
      }
      frame "---------- Macro ----------" {
        # "Do not put any code in this frame.\n(It is a separator no-op. You can make a copy of this frame to create a new Macro frame)"
        n154 = call <vilib>:"Add State(s) to Queue__jki_lib_state_machine.vi"("State(s) in (\"\")"=w394) -> ("States Out"=w393:string)  [unwired: 14 in]
      }
      frame "Macro: Setup Communications" {
        # "Exit Macro\n(This is called once, when the VI exits)"
        n155 = call <vilib>:"Add State(s) to Queue__jki_lib_state_machine.vi"("State(s) in Front (\"\")"="Connection: Init Status Connection EC\nConnection: Init Command Connection EC\nConnection: Init Status Connection LB\nConnection: Init Command Connection LB") -> ("States Out"=w397:string)  [unwired: 14 in]
        n156 = call <vilib>:"Add State(s) to Queue__jki_lib_state_machine.vi"("State(s) in Front (\"\")"=w397, "State(s) in (\"\")"=w401) -> ("States Out"=w400:string)  [unwired: 13 in]
      }
      frame "Macro: Exit" {
        # "Exit Macro\n(This is called once, when the VI exits)"
        n157 = Unbundle By Name(w406) -> ("Core.Close Panel on Exit?"=w407:bool)
        n158 = Select(t="UI: Front Panel State >> Close", s=w407, f="") -> (s? t:f=w410:string)
        n159 = call <vilib>:"Add State(s) to Queue__jki_lib_state_machine.vi"("State(s) in (\"\")"=w410, "State(s) at Back (\"\")"="Data: Cleanup\nExit") -> ("States Out"=w412:string)  [unwired: 13 in]
        n160 = call <vilib>:"Add State(s) to Queue__jki_lib_state_machine.vi"("State(s) in Front (\"\")"=w412, "State(s) in (\"\")"=w404) -> ("States Out"=w405:string)  [unwired: 13 in]
      }
      frame "Macro: Initialize" {
        w415 = "Data: Initialize\nInitialize Core Data\nUI: Initialize\nUI: Front Panel State >> Open\nMacro: Setup Communications\nMain: Check GPM Mode"  # Data: Initialize Initialize Core Data UI: Initialize UI: Front Panel State >> Open Macro: Setup Communications Main: Check GPM Mode
        n161 = call <vilib>:"Add State(s) to Queue__jki_lib_state_machine.vi"("State(s) in Front (\"\")"=w415, "State(s) in (\"\")"=w417) -> ("States Out"=w418:string)  [unwired: 13 in]
        n162 = property on="Pump" class="Bool"("DisabledEnum"=T18."Disabled and Grayed Out" ("Disabled")) -> ()  [unwired: 2 in, 2 out]
      }
      frame "---------- Main: Pre GPM Check----------" {
        # "Template Separator\n(You can make a copy of, or modify, this frame)"
        n163 = call <vilib>:"Add State(s) to Queue__jki_lib_state_machine.vi"("State(s) in (\"\")"=w423) -> ("States Out"=w422:string)  [unwired: 14 in]
      }
      frame "Main: Check GPM Mode" {
        n164 = Unbundle By Name(w432) -> ("GPM Mode"=w431:T1)
        n165 = Equal?(x=w431, y=GPM_Mode_typdef."Complete Global Pump Mode" ("GPM Mode")) -> (x = y?=w429:bool)
